vi "Perdite da termica.vi"(9 "Perdite da prova a vuoto 2":T1, 10 "Acqisizioni termica":T2, 11 "Ko - correz temp":dbl) -> (0 "Scorr 0":dbl, 2 "Perdite da termica":T3)   [LabVIEW 2019]
panel:
  # "PERDITE A CARICO"
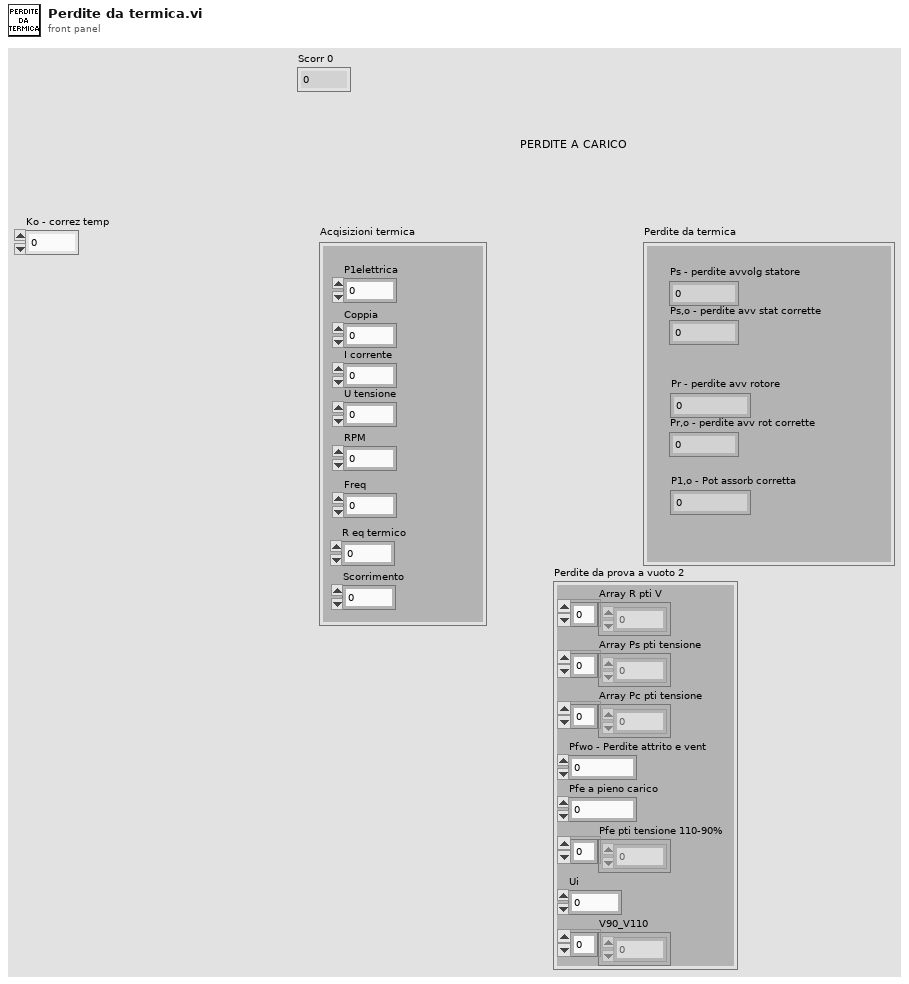
[diagram p1: front panel]
types:
  T1 = cluster{"Array R pti V":dbl[], "Array Ps pti tensione":dbl[], "Array Pc pti tensione":dbl[], "Pfwo - Perdite attrito e vent":dbl, "Pfe a pieno carico":dbl, "Pfe pti tensione 110-90% ":dbl[], "Ui":dbl, "V90_V110":dbl[]}
  T2 = cluster{"P1elettrica":dbl, "Coppia":dbl, "I corrente":dbl, "U tensione":dbl, "RPM":dbl, "Freq":dbl, "R eq termico":dbl, "Scorrimento":dbl}
  T3 = cluster{"Ps - perdite avvolg statore":dbl, "Ps,o - perdite avv stat corrette":dbl, "Pr - perdite avv rotore":dbl, "Pr,o - perdite avv rot corrette":dbl, "P1,o - Pot assorb corretta":dbl}
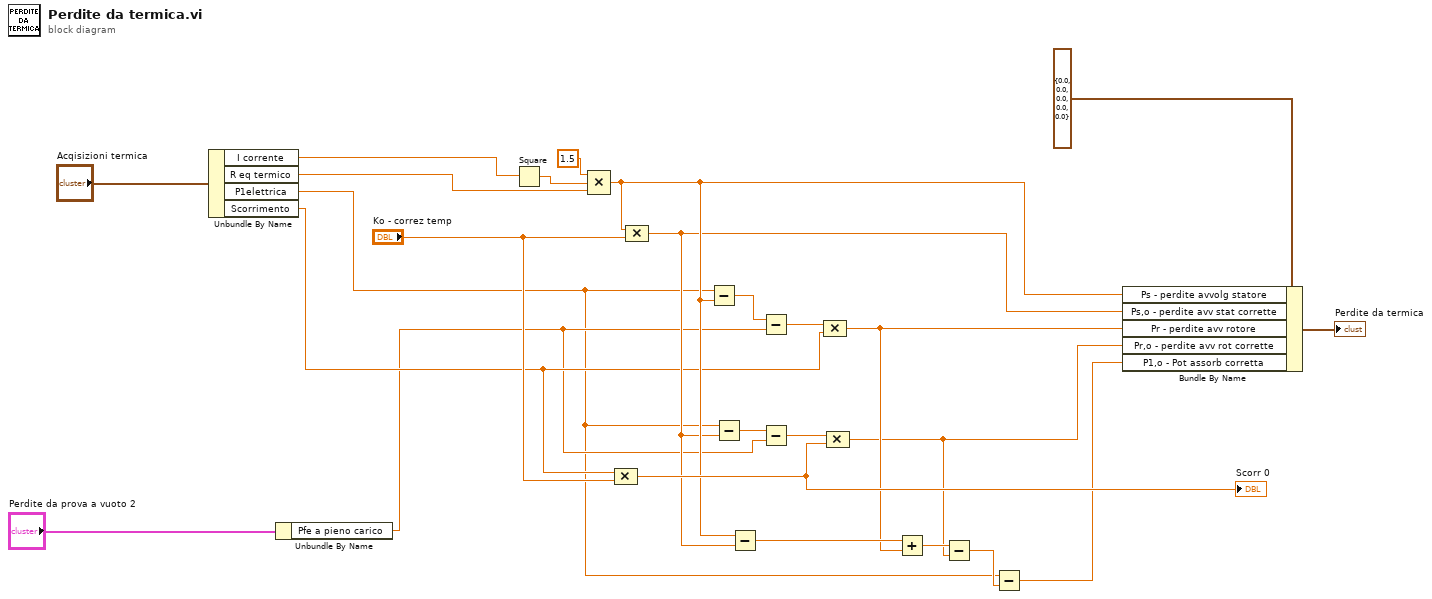
[diagram p0: block diagram]
diagram:
  n1 = Unbundle By Name("Acqisizioni termica") -> ("I corrente"=w7:dbl, "R eq termico"=w6:dbl, "P1elettrica"=w3:dbl, "Scorrimento"=w5:dbl)
  n2 = Unbundle By Name("Perdite da prova a vuoto 2") -> ("Pfe a pieno carico"=w4:dbl)
  n3 = Square(x=w7) -> (x^2=w25:dbl)
  n4 = Compound Arithmetic op=MULTIPLY(1.5 ("value"), w25, w6) -> (w13:dbl)
  n5 = Compound Arithmetic op=MULTIPLY(w5, "Ko - correz temp") -> (w18:dbl)
  "Scorr 0" <- w18
  n6 = Compound Arithmetic op=MULTIPLY(w13, "Ko - correz temp") -> (w12:dbl)
  n7 = Subtract(x=w3, y=w13) -> (x-y=w23:dbl)
  n8 = Subtract(x=w3, y=w12) -> (x-y=w21:dbl)
  n9 = Subtract(x=w13, y=w12) -> (x-y=w17:dbl)
  n10 = Subtract(x=w23, y=w4) -> (x-y=w22:dbl)
  n11 = Subtract(x=w21, y=w4) -> (x-y=w20:dbl)
  n12 = Compound Arithmetic op=MULTIPLY(w22, w5) -> (w11:dbl)
  n13 = Compound Arithmetic op=MULTIPLY(w20, w18) -> (w2:dbl)
  n14 = Add(x=w17, y=w11) -> (x+y=w16:dbl)
  n15 = Subtract(x=w16, y=w2) -> (x-y=w15:dbl)
  n16 = Subtract(x=w3, y=w15) -> (x-y=w10:dbl)
  n17 = Bundle By Name(cluster=T3 {"Ps - perdite avvolg statore"=0.0, "Ps,o - perdite avv stat corrette"=0.0, "Pr - perdite avv rotore"=0.0, "Pr,o - perdite avv rot corrette"=0.0, "P1,o - Pot assorb corretta"=0.0} ("Cluster"), "Ps - perdite avvolg statore"=w13, "Ps,o - perdite avv stat corrette"=w12, "Pr - perdite avv rotore"=w11, "Pr,o - perdite avv rot corrette"=w2, "P1,o - Pot assorb corretta"=w10) -> (→"Perdite da termica":T3)
